vi "Read Mouse.vi"(8 "error in (no error)":errorcluster, 11 "Picture.lvclass in":refnum<class "Picture.lvclass">) -> (0 "error out":errorcluster, 2 "Mouse":T1, 3 "Picture.lvclass out":refnum<class "Picture.lvclass">)   [LabVIEW 2015, in "Picture.lvclass"]
uses:
  Picture.lvclass
  <vilib>/Utility/miscctls.llb/LVMouseTypeDef.ctl
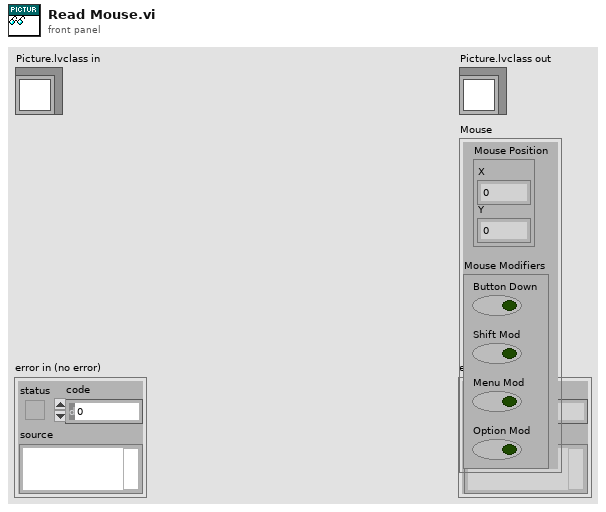
[diagram p1: front panel]
types:
  T1 = typedef "LVMouseTypeDef.ctl" = cluster{"Mouse Position":cluster{"X":i32, "Y":i32}, "Mouse Modifiers":cluster{"Button Down":bool, "Shift Mod":bool, "Menu Mod":bool, "Option Mod":bool}}
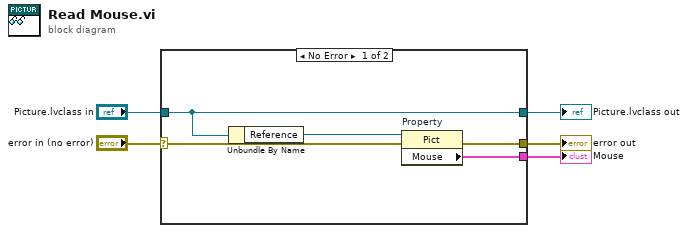
[diagram p0: block diagram]
diagram:
  n1 = case shown="No Error" "error in (no error)" {
    selector: "error in (no error)" -> [w6 w12]
    tunnel: [w9 w12] -> w4
    tunnel: [w8 w11] -> w2
    tunnel: "Picture.lvclass in" -> [w8 w11]
    tunnel: [w10 _] -> w1
    frame No Error {
      n2 = Unbundle By Name(w8) -> ("Reference"=w7:refnum<vi>)
      n3 = property on="Property" class="Pict"(reference=w7, error in=w6) -> (error out=w9:errorcluster, "Mouse"=w10:T1)  [unwired: 1 out]
    }
    frame Error {
    }
  }
  "error out" <- w4
  "Picture.lvclass out" <- w2
  "Mouse" <- w1
